vi "Actor Teardown.vi"(10 "Error":errorcluster, 11 "Dev Actor in":refnum<class "Dev Actor.lvclass">) -> (0 "error out":errorcluster, 2 "Teardown?":bool, 3 "Dev Actor out":refnum<class "Dev Actor.lvclass">)   [LabVIEW 2021, in "Dev Actor.lvlib" / "Dev Actor.lvclass"]
uses:
  Dev Actor.lvclass
  Dev Actor.lvclass/Dev Actor.ctl
  Panel/Panel.lvclass
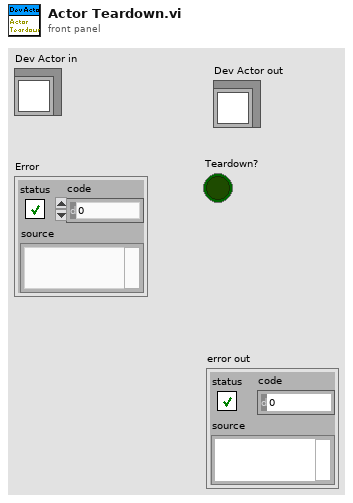
[diagram p1: front panel]
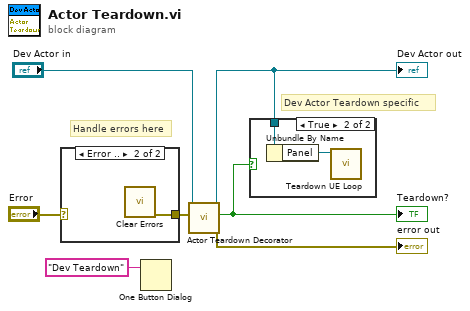
[diagram p0: block diagram]
diagram:
  # "Dev Actor Teardown specific"
  # "Handle errors here"
  n1 = case shown="Error .." "Error" {
    tunnel: [_ w8] -> w5
    frame No Error {
    }
    frame Error {
      n2 = call <vilib>:"Clear Errors.vi"() -> ("error out"=w8:errorcluster)  [unwired: 6 in, 1 out]
    }
  }
  n3 = One Button Dialog(message="Dev Teardown") -> ()  [unwired: 1 in, 1 out]
  n4 = call "Actor Teardown Decorator.vi"("Error"=w5, "Dev Actor in"="Dev Actor in") -> ("error out"=→"error out":errorcluster, "Teardown?"=w3:bool, "Dev Actor out"=w1:refnum<class "Dev Actor.lvclass">)  [unwired: 7 in]
  "Teardown?" <- w3
  "Dev Actor out" <- w1
  n5 = case shown="True" w3 {
    tunnel: w1 -> [_ w10]
    frame False {
    }
    frame True {
      n6 = Unbundle By Name(w10) -> ("Panel"=w9:refnum<class "Panel.lvclass">)
      n7 = call-dynamic "Teardown UE Loop.vi"("Panel in"=w9) -> ()  [unwired: 10 in, 1 out]
    }
  }
